vi "initialise.vi"(8 "error in (no error)":errorcluster, 11 "k3390_AWG in":refnum<class "k3390_AWG.lvclass">) -> (0 "error out":errorcluster, 3 "k3390_AWG out":refnum<class "k3390_AWG.lvclass">)   [LabVIEW 2009, in "Hardware.lvlib" / "Channels.lvlib" / "k3390_AWG.lvclass"]
uses:
  k3390_AWG.lvclass
  k3390_AWG.lvclass/k3390_AWG.ctl
  <instrlib>/Keithley 3390/Keithley 3390.lvlib
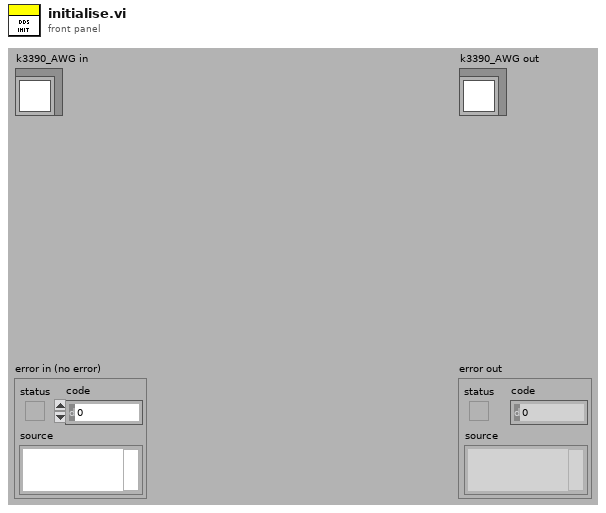
[diagram p1: front panel]
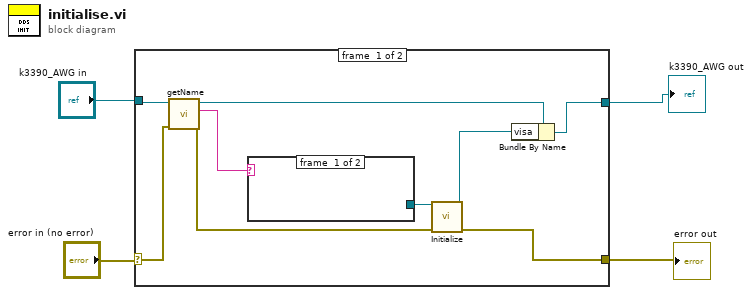
[diagram p0: block diagram]
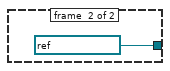
[diagram p2: hidden frame]
diagram:
  n1 = case shown="No Error" "error in (no error)" {
    selector: "error in (no error)" -> [w12 w15]
    tunnel: "k3390_AWG in" -> [w13 w16]
    tunnel: [w6 w15] -> w1
    tunnel: [w5 w16] -> w2
    frame #0 {
      n2 = call-dynamic "getName.vi"("error in (no error)"=w12, "DDSOutput in"=w13) -> ("error out"=w9:errorcluster, "name"=w10:string, "DDSOutput out"=w8:refnum<class "k3390_AWG.lvclass">)  [unwired: 7 in]
      n3 = case shown="\"k3390\"" w10 {
        tunnel: [_ refnum<visa-resource-name> "k3390" ("VISA resource name")] -> w11
        frame #0 {
        }
        frame #1 {
        }
      }
      n4 = call <instrlib>:"Initialize.vi"("error in (no error)"=w9, "VISA resource name"=w11) -> ("error out"=w6:errorcluster, "VISA resource name out"=w7:refnum<visa-resource-name>)  [unwired: 8 in]
      n5 = Bundle By Name(cluster=w8, "visa"=w7) -> (w5:refnum<class "k3390_AWG.lvclass">)
    }
    frame #1 {
    }
  }
  "error out" <- w1
  "k3390_AWG out" <- w2
